vi "LVClass_CorrectionDataManager GetDiagnosticsEigenVector.vi"(0 "CorrectionDataManager in":refnum<class "CorrectionDataManager.lvclass">, 5 "n° mode":i32, 9 "HasoSlopes in":refnum<class "HasoSlopes.lvclass">, 11 "error in (no error)":errorcluster) -> (4 "CorrectionDataManager out":refnum<class "CorrectionDataManager.lvclass">, 8 "commands":sgl[](array[numeric]), 10 "HasoSlopes out":refnum<class "HasoSlopes.lvclass">, 15 "error out":errorcluster)   [LabVIEW 2020, in "CorrectionDataManager.lvclass"]
doc: "Get HasoSlopes object and commands array associated to an influence.\n\n<B>corrdata_managerIn</B> : CorrDataManager object.\n<B>corrdata_managerOut</B> : CorrDataManager object.\n<B>mode_index</B> : Influence index.\n<B>right_eigenvector</B> : HasoSlopes or Phase object.\n<B>commands</B> : Command array .\n<B>is_phase</B> : define if right_eigenvector container is a HasoSlopes or Phase."
uses:
  CorrectionDataManager.lvclass
  HasoSlopes/HasoSlopes.lvclass
  CorrectionDataManager.lvclass/CorrectionDataManager.ctl
  HasoSlopes/LVClass_HasoSlopes Read HasoSlopes _ property.vi
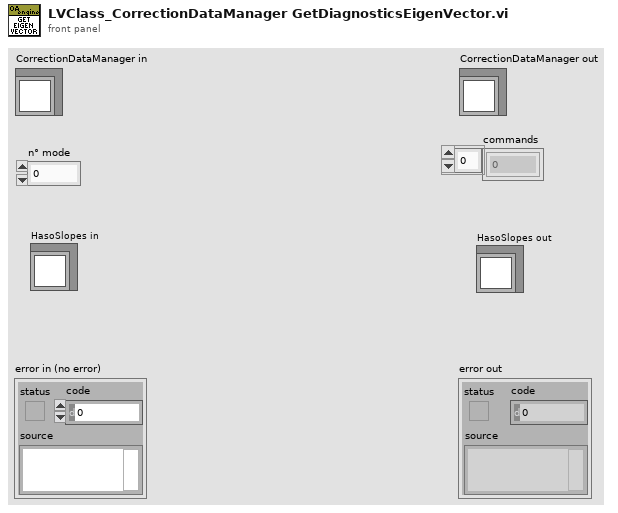
[diagram p1: front panel]
types:
  T1 = typedef "ClassID.ctl" = i64
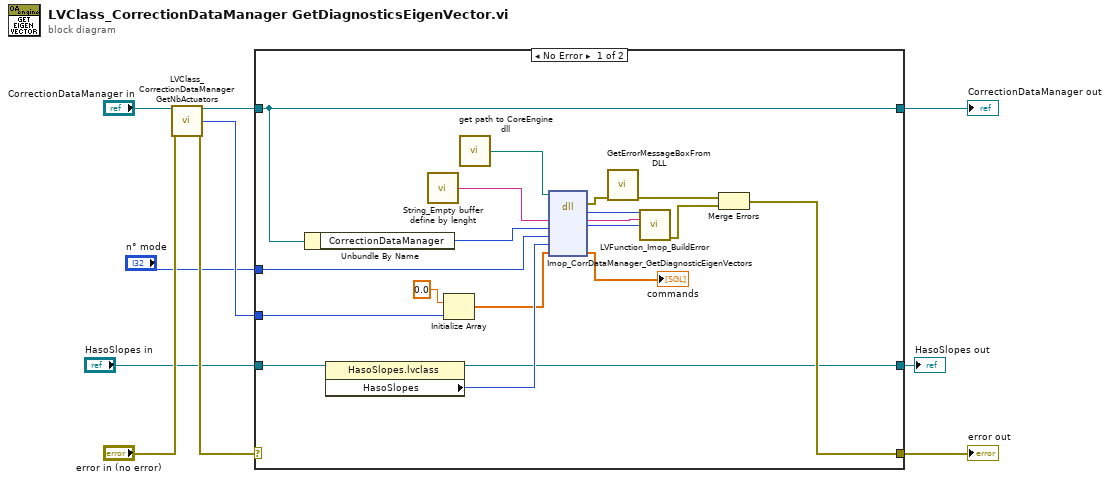
[diagram p0: block diagram]
diagram:
  n1 = call "LVClass_CorrectionDataManager GetNbActuators.vi"("CorrectionDataManager in"="CorrectionDataManager in", "error in (no error)"="error in (no error)") -> ("CorrectionDataManager out"=w7:refnum<class "CorrectionDataManager.lvclass">, "Nb actuators"=w6:i32, "error out"=w4:errorcluster)  [unwired: 11 in]
  n2 = case shown="No Error" w4 {
    selector: w4 -> [_ w32]
    tunnel: [w23 w32] -> w9
    tunnel: [w20 w31] -> w10
    tunnel: w7 -> [w20 w31]
    tunnel: w6 -> [w18 _]
    tunnel: "n° mode" -> [w17 _]
    tunnel: "HasoSlopes in" -> [w16 w30]
    tunnel: [w14 w30] -> w1
    frame No Error {
      n3 = Unbundle By Name(w20) -> ("CorrectionDataManager"=w19:T1)
      n4 = property class="HasoSlopes.lvclass"(reference=w16) -> (reference out=w14:refnum<class "HasoSlopes.lvclass">, "HasoSlopes"=w15:T1)  [unwired: 1 in, 1 out]
      n5 = call "String_Empty buffer define by lenght.vi"() -> ("Empty buffer"=w27:string)  [unwired: 1 in]
      n6 = Initialize Array(sgl 0.0, w18) -> (w13:sgl[])
      n7 = call "get path to CoreEngine dll.vi"() -> ("path to wavekit library"=w21:path)  [unwired: 14 in, 1 out]
      n8 = dll-call lib="D:/soft/HASO_v3/SVN_trunk/ImOpCoreEngine4_LV2011/DLLs/c_interface_vc100.dll" fn="Imop_CorrDataManager_GetDiagnosticEigenVectors"(path in=w21, "message"=w27, "corrdata_manager"=w19, "n° mode"=w17, "HasoSlopes"=w15, "commands"=w13) -> (error out=w26:errorcluster, "return type"=w29:i32, "message"=w28:string, "corrdata_manager"=w11:i64, "commands"=→"commands":sgl[])  [unwired: 4 in, 1 out]
      n9 = call "GetErrorMessageBoxFromDLL.vi"("error IN"=w26) -> ("error OUT"=w25:errorcluster)  [unwired: 10 in]
      n10 = call "LVFunction_Imop_BuildError.vi"("code"=w29, "String to Prepend to source (\"\")"=w28, "Adresse"=w11) -> ("error out"=w24:errorcluster)  [unwired: 12 in]
      n11 = Merge Errors(w25, w24) -> (w23:errorcluster)
    }
    frame Error {
    }
  }
  "error out" <- w9
  "CorrectionDataManager out" <- w10
  "HasoSlopes out" <- w1
